vi "Add Items.vi"(4 "indent":i32, 6 "Insertion index":i32, 8 "error in (no error)":errorcluster, 10 "Items to Add":refnum<class "BetterItem.lvclass">[](array[class]), 11 "Better Tree Handle In":refnum<class "BetterTreeHandle.lvclass">) -> (0 "error out":errorcluster, 3 "Better Tree Handle Out":refnum<class "BetterTreeHandle.lvclass">)   [LabVIEW 2020, in "BetterDragAndDrop.lvlib" / "BetterTreeHandle.lvclass"]
uses:
  BetterTreeHandle.lvclass
  C:/DSCE code/Open-source/betterdraganddrop_GIT/Source/Classes/BetterHandle/BetterHandle.lvclass
  BetterTreeItem/BetterItem.lvclass
  BetterHandle/BetterHandle.lvclass/BetterHandle.ctl
  BetterTreeHandle.lvclass/BetterTreeHandle.ctl
  BetterTreeItem/SubVIs/Re-Anchor steps TreeItemObjs.vi
  BetterHandle/BetterHandle.lvclass
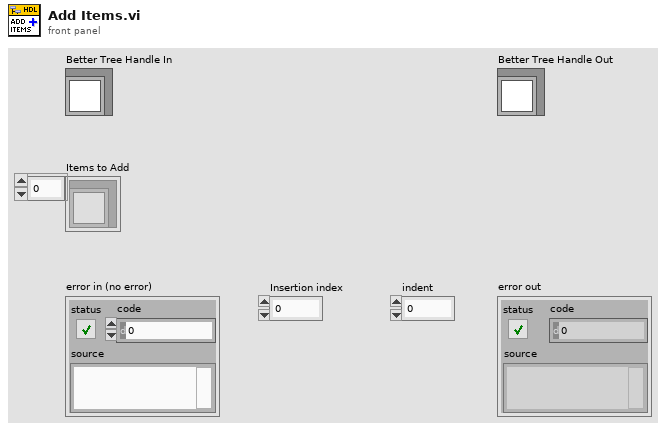
[diagram p1: front panel]
types:
  T1 = typedef "BetterDragAndDrop.lvlib/BetterTreeHandle.lvclass/TreeItem.ctl" = cluster{"Left Cell String":string, "Child Text":string[], "Child Tag":string, "Item Indent":i32, "Child Only?":bool, "Glyph Index":i32, "Font Color":u32}
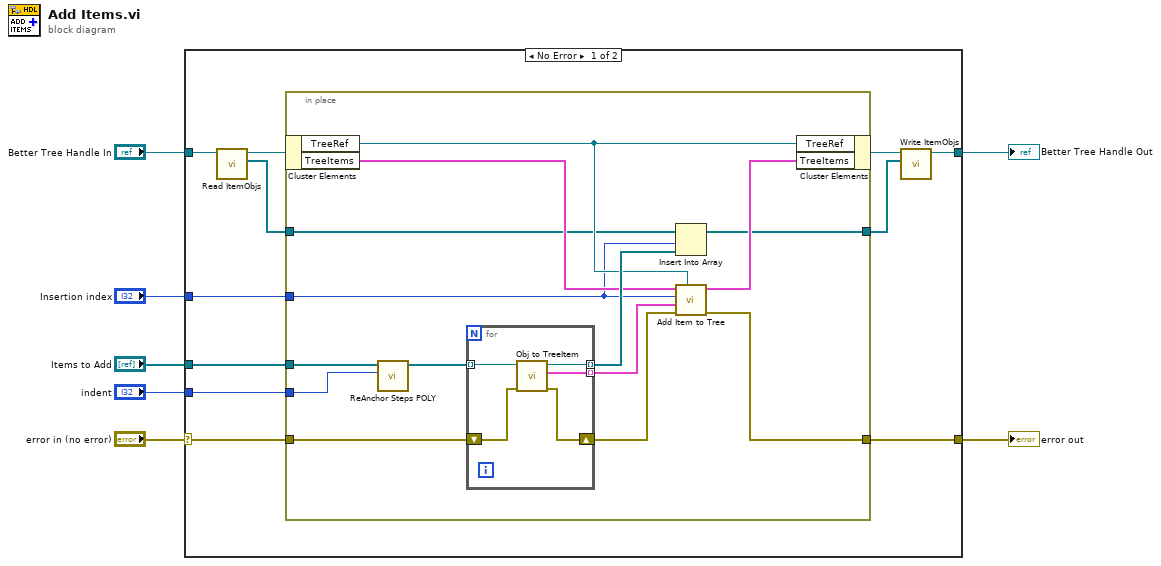
[diagram p0: block diagram]
diagram:
  n1 = case shown="No Error" "error in (no error)" {
    selector: "error in (no error)" -> [w17 w39]
    tunnel: [w18 w39] -> w7
    tunnel: "indent" -> [w16 _]
    tunnel: "Insertion index" -> [w15 _]
    tunnel: "Better Tree Handle In" -> [w13 w38]
    tunnel: [w9 w38] -> w2
    tunnel: "Items to Add" -> [w14 _]
    frame No Error {
      n2 = call "Read ItemObjs.vi"("BetterHandle in"=w13) -> ("ItemObjs"=w11:refnum<class "BetterItem.lvclass">[], "BetterHandle out"=w12:refnum<class "BetterTreeHandle.lvclass">)  [unwired: 9 in]
      n3 = in-place {
        in-place-border: w14 -> [w21]
        in-place-border: w17 -> [w31]
        in-place-border: [w26] -> w18
        in-place-border: w16 -> [w23]
        in-place-border: w15 -> [w24]
        in-place-border: w11 -> [w20]
        in-place-border: [w19] -> w8
        n4 = in-place-cluster #1(w12) -> ("TreeRef"=w25:refnum<vi>, "TreeItems"=w30:T1[])
        n5 = call-poly "ReAnchor Steps POLY.vi"("indent (i=0)"=w23, "TreeItemObjs"=w21) -> ("TreeItemObjs"=w22:refnum<class "BetterItem.lvclass">[])  [unwired: 9 in]
        n6 = for {
          tunnel: w22 -> [w37] mode=indexing
          tunnel: [w34] -> w32 mode=indexing
          tunnel: [w33] -> w29 mode=indexing
          shift-right: [w35] -> w27
          shift-left: w31 -> [w36]
          n7 = call "Obj to TreeItem.vi"("error in (no error)"=w36, "BetterTreeItem in"=w37) -> ("error out"=w35:errorcluster, "Tree Control Item"=w33:T1, "BetterTreeItem out"=w34:refnum<class "BetterItem.lvclass">)  [unwired: 7 in]
        }
        n8 = Insert Into Array(array=w20, index=w24, new element=w32) -> (w19:refnum<class "BetterItem.lvclass">[])
        n9 = call "Add Item to Tree.vi"("Tree ref"=w25, "error in (no error)"=w27, "TreeItems (to add)"=w29, "Insertion index"=w24, "TreeItems (current)"=w30) -> ("error out"=w26:errorcluster, "TreeItems (added)"=w28:T1[])  [unwired: 5 in]
        n10 = in-place-cluster #1("TreeRef"=w25, "TreeItems"=w28) -> (w10:refnum<class "BetterTreeHandle.lvclass">)
      }
      n11 = call "Write ItemObjs.vi"("ItemObjs"=w8, "BetterHandle in"=w10) -> ("BetterHandle out"=w9:refnum<class "BetterTreeHandle.lvclass">)  [unwired: 9 in]
    }
    frame Error {
    }
  }
  "error out" <- w7
  "Better Tree Handle Out" <- w2
